vi "Close Device.vi"(8 "error in (no error)":errorcluster, 11 "Device in":refnum<class "PIC-Device.lvclass">) -> (0 "error out":errorcluster, 3 "Device out":refnum<class "PIC-Device.lvclass">)   [LabVIEW 2020, in "PIC-Device.lvclass"]
doc: "Closes the device"
uses:
  PIC-Device.lvclass
  Instruments/Power Supply/Power Supply.lvclass
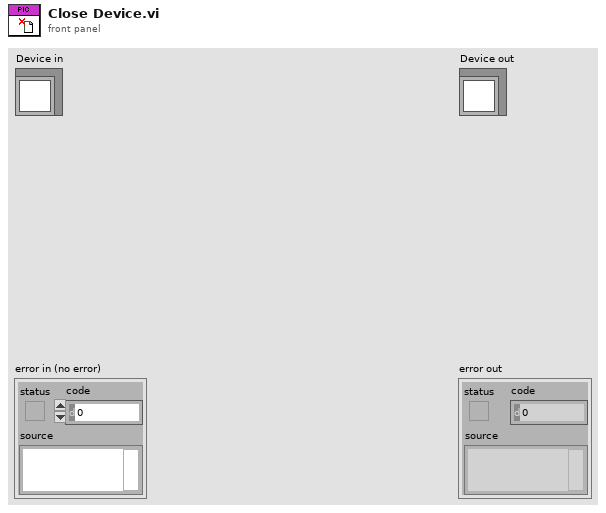
[diagram p1: front panel]
types:
  T1 = typedef "Device.lvclass/DC Offset Cluster.ctl" = cluster{"Enable":bool, "Use Array":bool, "Array":dbl[], "To From Cluster":cluster{"From":dbl, "To":dbl, "Step":dbl}, "Current Value":dbl, "DC Offset":refnum<class "Power Supply.lvclass">}
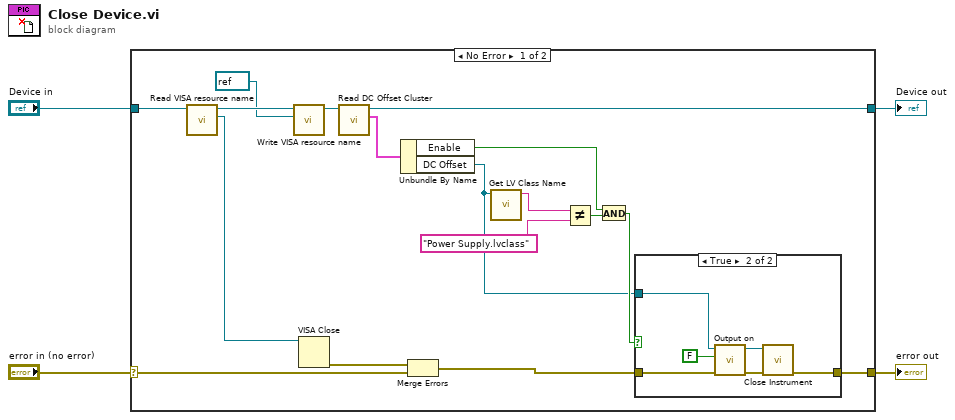
[diagram p0: block diagram]
diagram:
  n1 = case shown="No Error" "error in (no error)" {
    selector: "error in (no error)" -> [w7 w30]
    tunnel: [w13 w30] -> w3
    tunnel: [w8 w29] -> w1
    tunnel: "Device in" -> [w12 w29]
    frame No Error {
      n2 = call-dynamic "Read VISA resource name.vi"("Device in"=w12) -> ("VISA resource name"=w21:refnum<visa-resource-name>, "Device out"=w10:refnum<class "PIC-Device.lvclass">)  [unwired: 9 in]
      n3 = call-dynamic "Write VISA resource name.vi"("VISA resource name"=refnum<visa-resource-name> refnum, "Device in"=w10) -> ("Device out"=w11:refnum<class "PIC-Device.lvclass">)  [unwired: 9 in]
      n4 = VISA Close(VISA resource name=w21) -> (error out=w6:errorcluster)  [unwired: 1 in]
      n5 = call-dynamic "Read DC Offset Cluster.vi"("Device in"=w11) -> ("DC Offset Cluster"=w20:T1, "Device out"=w8:refnum<class "PIC-Device.lvclass">)  [unwired: 8 in, 1 out]
      n6 = Unbundle By Name(w20) -> ("Enable"=w16:bool, "DC Offset"=w14:refnum<class "Power Supply.lvclass">)
      n7 = Merge Errors(w6, w7) -> (w5:errorcluster)
      n8 = call <vilib>:"Get LV Class Name.vi"("object"=w14) -> ("class name"=w19:string)  [unwired: 9 in, 1 out]
      n9 = Not Equal?(x=w19, y="Power Supply.lvclass") -> (x != y?=w17:bool)
      n10 = And(x=w16, y=w17) -> (x .and. y?=w15:bool)
      n11 = case shown="True" w15 {
        tunnel: w14 -> [_ w28]
        tunnel: w5 -> [w22 w26]
        tunnel: [w22 w23] -> w13
        frame False {
        }
        frame True {
          n12 = call-dynamic "Output on.vi"("error in (no error)"=w26, "Output On"=FALSE, "Power Supply in"=w28) -> ("error out"=w25:errorcluster, "Power Supply out"=w24:refnum<class "Power Supply.lvclass">)  [unwired: 7 in]
          n13 = call-dynamic "Close Instrument.vi"("error in (no error)"=w25, "Instrument in"=w24) -> ("error out"=w23:errorcluster)  [unwired: 8 in, 1 out]
        }
      }
    }
    frame Error {
    }
  }
  "error out" <- w3
  "Device out" <- w1
